vi "AP_project_calibration.vi"() -> ()   [LabVIEW 2019]
uses:
  <vilib>/userDefined/High Color/IMAQdx.ctl
  <vilib>/vision/driver/IMAQdx.llb/IMAQdx Acquisition Mode.ctl
  <vilib>/vision/driver/IMAQdx.llb/IMAQdx Buffer Number Mode.ctl
  <vilib>/vision/driver/NI_Vision_Acquisition_Software.lvlib
  <vilib>/vision/NI_Vision_Development_Module.lvlib
panel:
  in  "Range":cluster{"Lower value":sgl, "Upper value":sgl}={"Lower value"=50.0, "Upper value"=140.0} {"Upper value" format="%.2f"; "Lower value" format="%.2f"}
  out "DisplayFrameRate":dbl(knob) scale=0.0..100.0 scale format="%.1f"
  in  "IMAQdx Session":T1="cam0"
  out "ProcessBufferNumber":u32
  out "ProcessFrameRate":dbl(knob) scale=0.0..100.0 scale format="%.1f"
  out "Processed Image":T2(plugin-control)
  out "# elements in queue":i32(knob) scale=0.0..250.0
  in  "stop":bool
  out "CameraFrameRate":dbl(knob) scale=0.0..100.0 scale format="%.1f"
  out "CameraBuffer Number":u32
  out "Acquired Image":T2(plugin-control)
  out "height":dbl
  out "width":dbl
  in  "Display Index":i32
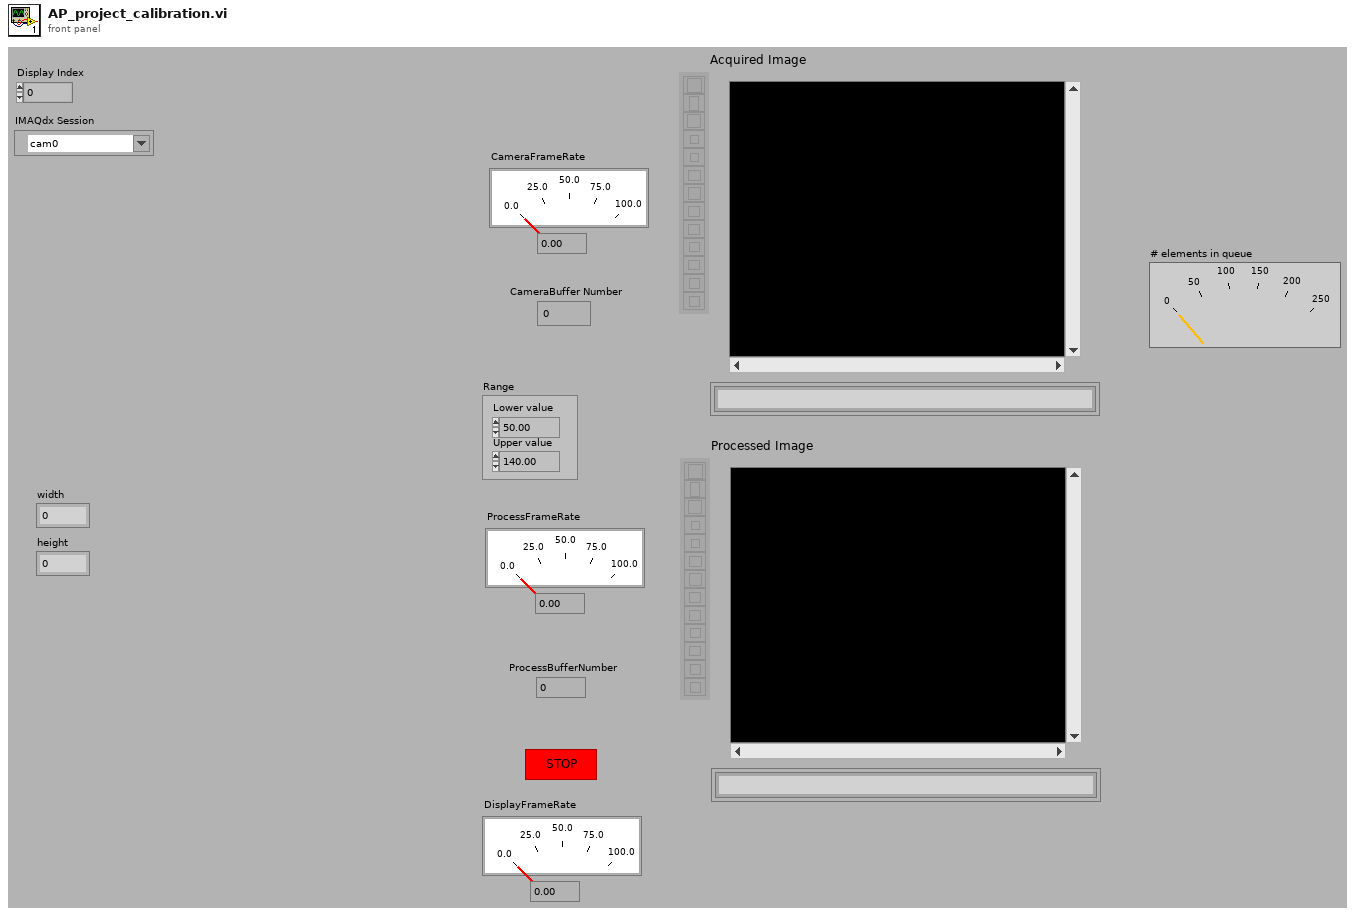
[diagram p1: front panel]
types:
  T1 = typedef "IMAQdx.ctl" = refnum<k21>
  T2 = typedef "IMAQ Image.ctl" = refnum<image>
  T3 = typedef "NI_Vision_Acquisition_Software.lvlib/IMAQdx Buffer Number Mode.ctl" = enum32{"Next", "Last", "Buffer Number", "Every", "Last New"}
  T4 = typedef "LVAllMonitorsDisplayTypeDef.ctl" = cluster{"Bounds":cluster{"Left":i16, "Top":i16, "Right":i16, "Bottom":i16}, "Depth":i16}[]
  T5 = cluster{"Bounds":cluster{"Left":i16, "Top":i16, "Right":i16, "Bottom":i16}, "Depth":i16}
  T6 = typedef "Image Type" = u32
  T7 = typedef "NI_Vision_Acquisition_Software.lvlib/IMAQdx Acquisition Mode.ctl" = enum32{"One Shot", "Continuous"}
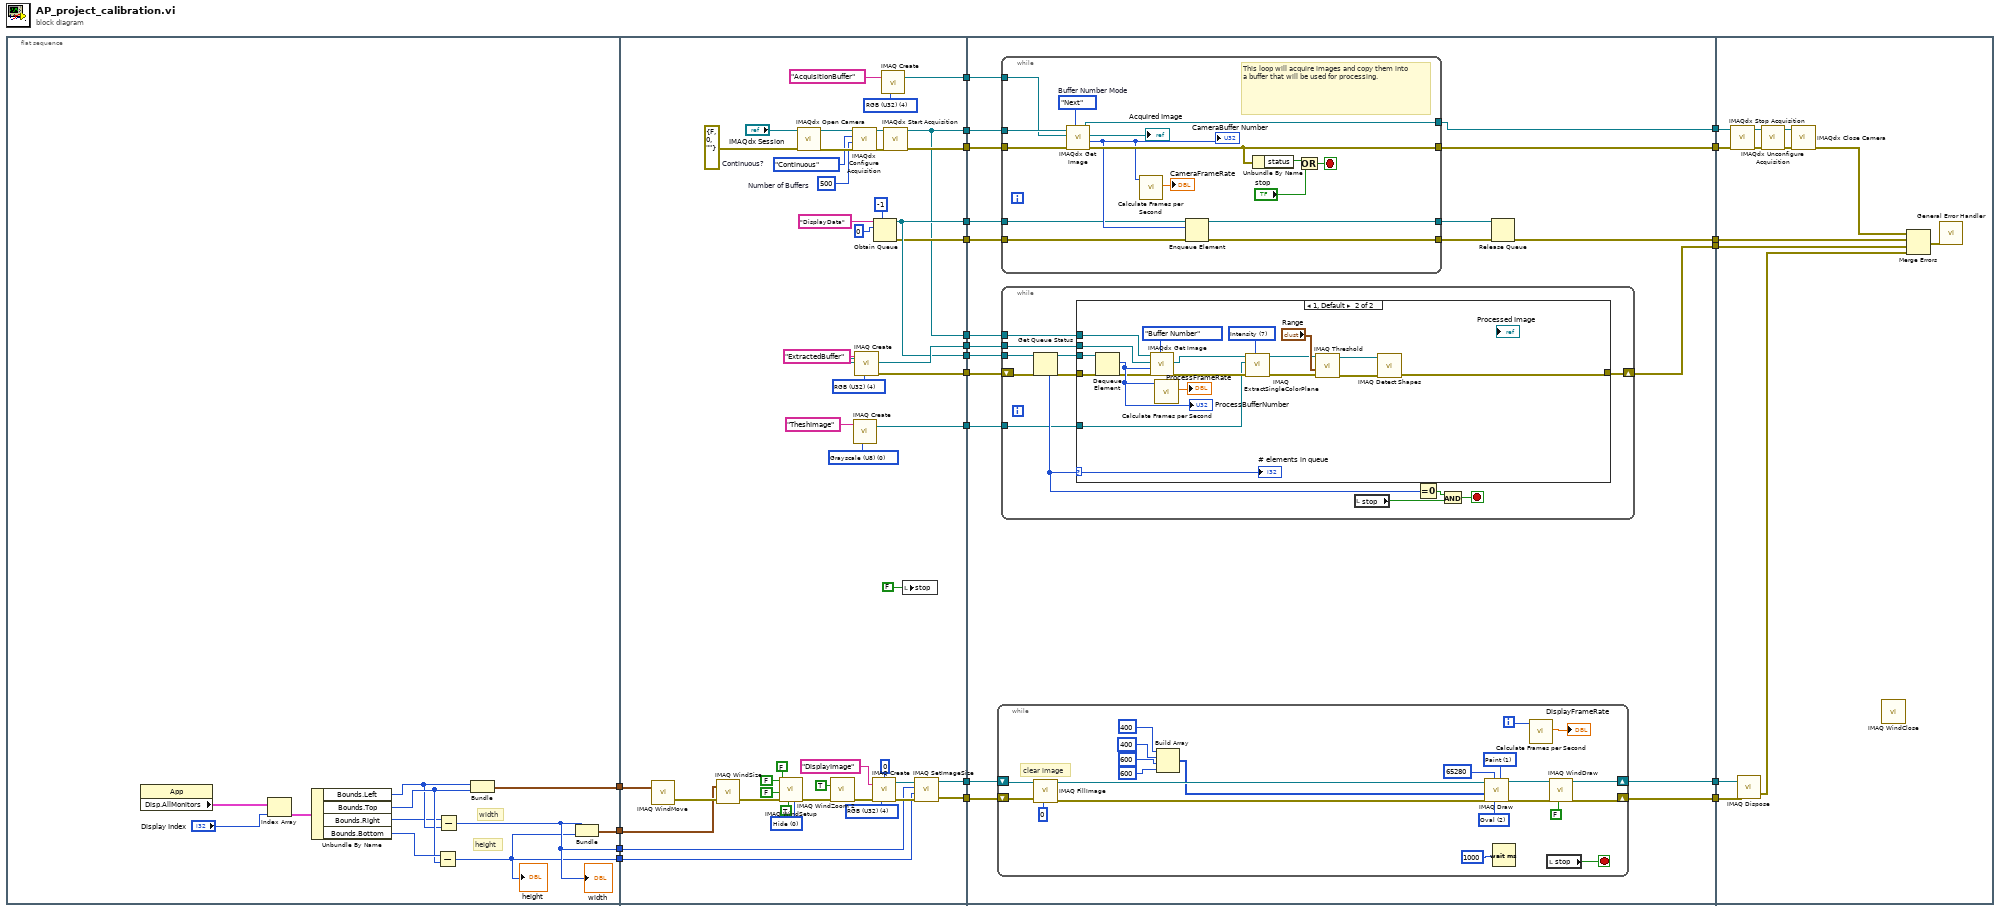
[diagram p0: block diagram]
diagram:
  n1 = flat-sequence {
    tunnel: [w26] -> w21
    tunnel: [w25] -> w20
    tunnel: [w24] -> w6
    tunnel: [w23] -> w5
    tunnel: [w45] -> w22
    tunnel: w21 -> [w77]
    tunnel: w20 -> [w75]
    tunnel: [w55] -> w19
    tunnel: [w54] -> w18
    tunnel: [w53] -> w17
    tunnel: [w53] -> w16
    tunnel: [w52] -> w15
    tunnel: [w51] -> w14
    tunnel: [w50] -> w9
    tunnel: [w50] -> w8
    tunnel: [w40] -> w7
    tunnel: w6 -> [w39]
    tunnel: w5 -> [w38]
    tunnel: [w37] -> w2
    tunnel: [w34] -> w1
    tunnel: w22 -> [w100]
    tunnel: w19 -> [w97]
    tunnel: w18 -> [w96]
    tunnel: w17 -> [w95]
    tunnel: w16 -> [w94]
    tunnel: w15 -> [w93]
    tunnel: w14 -> [w92]
    tunnel: [w91] -> w13
    tunnel: [w90] -> w12
    tunnel: [w89] -> w11
    tunnel: [w88] -> w10
    tunnel: w9 -> [w87]
    tunnel: w8 -> [w86]
    tunnel: w7 -> [w85]
    tunnel: [w84] -> w4
    tunnel: [w83] -> w3
    tunnel: w2 -> [w82]
    tunnel: w1 -> [w81]
    tunnel: w13 -> [w182]
    tunnel: w12 -> [w181]
    tunnel: w11 -> [w176]
    tunnel: w10 -> [w175]
    tunnel: w4 -> [w173]
    tunnel: w3 -> [w172]
    frame #0 {
      # "height"
      # "width"
      n2 = property class="App"() -> ("Disp.AllMonitors"=w29:T4)  [unwired: 2 in, 2 out]
      n3 = Index Array(array=w29, index="Display Index") -> (element=w28:T5)
      n4 = Unbundle By Name(w28) -> ("Bounds.Left"=w31:i16, "Bounds.Top"=w32:i16, "Bounds.Right"=w30:i16, "Bounds.Bottom"=w33:i16)
      n5 = Subtract(x=w33, y=w32) -> (x-y=w23:i16)
      "height" <- w23
      n6 = Subtract(x=w30, y=w31) -> (x-y=w24:i16)
      "width" <- w24
      n7 = Bundle("Left"=w31, "Top"=w32) -> (w25:cluster{"Left":i16, "Top":i16})  [unwired: 1 in]
      n8 = Bundle(w24, w23) -> (w26:cluster{i16, i16})  [unwired: 1 in]
    }
    frame #1 {
      w35 = T6 0 items=["Grayscale (U8)", "Grayscale (I16)", "Grayscale (SGL)", "Complex (CSG)", "RGB (U32)", "HSL (U32)", "RGB (U64)"] ("Image Type")
      w41 = T6 4 items=["Grayscale (U8)", "Grayscale (I16)", "Grayscale (SGL)", "Complex (CSG)", "RGB (U32)", "HSL (U32)", "RGB (U64)"] ("Image Type")
      w63 = T6 4 items=["Grayscale (U8)", "Grayscale (I16)", "Grayscale (SGL)", "Complex (CSG)", "RGB (U32)", "HSL (U32)", "RGB (U64)"] ("Image Type")
      w56 = T6 4 items=["Grayscale (U8)", "Grayscale (I16)", "Grayscale (SGL)", "Complex (CSG)", "RGB (U32)", "HSL (U32)", "RGB (U64)"] ("Image Type")
      w62 = u32 500  # Number of Buffers
      w61 = IMAQdx_Acquisition_Mode."Continuous"  # Continuous?
      w74 = 0 items=["Hide", "Show", "No change"] ("Scrollbars (No change)")
      n9 = call "IMAQ WindMove"("Coordinates (screen)"=w75) -> ("error out"=w79:errorcluster)  [unwired: 4 in, 1 out]
      n10 = call "IMAQ WindSize"("error in (no error)"=w79, "Width & Height"=w77) -> ("error out"=w80:errorcluster)  [unwired: 4 in, 2 out]
      n11 = call "IMAQ WindSetup"("Scrollbars (No change)"=w74, "Window is floating? (No)"=TRUE, "error in (no error)"=w80, "Window has title bar? (Yes)"=FALSE, "Window can close? (Yes)"=FALSE, "Window can grow? (Yes)"=FALSE) -> ("error out"=w78:errorcluster)  [unwired: 5 in]
      n12 = call <vilib>:"IMAQdx Open Camera.vi"("error in"=errorcluster {"status"=FALSE, "code"=0, "source"=""}, "Session In"="IMAQdx Session") -> ("error out"=w68:errorcluster, "Session Out"=w69:T1)  [unwired: 8 in]
      n13 = call "IMAQ WindZoom 2"("error in (no error)"=w78, "Zoom to Fit? (False)"=TRUE ("Zoom to Fit? (T)")) -> ("error out"=w44:errorcluster)  [unwired: 6 in, 3 out]
      n14 = call <vilib>:"IMAQdx Configure Acquisition.vi"("error in"=w68, "Number of Buffers"=w62, "Continuous?"=w61, "Session In"=w69) -> ("error out"=w67:errorcluster, "Session Out"=w65:T1)  [unwired: 6 in]
      n15 = call "IMAQ Create"("Image Name"="TheshImage", "Image Type"=w35) -> ("New Image"=w34:T2)  [unwired: 3 in, 1 out]
      n16 = call "IMAQ Create"("Image Name"="ExtractedBuffer", "Image Type"=w63) -> ("New Image"=w55:T2, "error out"=w37:errorcluster)  [unwired: 3 in]
      n17 = call "IMAQ Create"("Border Size"=0, "Image Name"="DisplayImage", "Image Type"=w41, "error in (no error)"=w44) -> ("New Image"=w46:T2, "error out"=w47:errorcluster)  [unwired: 1 in]
      n18 = Obtain Queue(max queue size (-1, unlimited)=-1, name (unnamed)="DisplayData", element data type=u32 0) -> (queue out=w53:refnum<queue>, error out=w52:errorcluster)  [unwired: 2 in, 1 out]
      n19 = call "IMAQ Create"("Image Name"="AcquisitionBuffer", "Image Type"=w56) -> ("New Image"=w51:T2)  [unwired: 3 in, 1 out]
      n20 = call <vilib>:"IMAQdx Start Acquisition.vi"("error in"=w67, "Session In"=w65) -> ("error out"=w54:errorcluster, "Session Out"=w50:T1)  [unwired: 8 in]
      n21 = local write "stop"(FALSE ("stop")) -> ()
      n22 = call "IMAQ SetImageSize"("error in (no error)"=w47, "Y Resolution"=w38, "X Resolution"=w39, "Image"=w46) -> ("error out"=w45:errorcluster, "Image Out"=w40:T2)  [unwired: 1 in]
    }
    frame #2 {
      n23 = while {
        shift-right: [w164] -> w84
        shift-left: w85 -> [w168]
        shift-right: [w163] -> w83
        shift-left: w100 -> [w167]
        i -> [w162]
        stop <- w169 stop-if-true
        w157 = u16 1 items=["Frame", "Paint", "Invert Frame", "Invert Paint"] ("Draw Mode")
        w156 = u16 2 items=["Line", "Rectangle", "Oval"] ("Shape to draw")
        # "clear image"
        n24 = call "IMAQ FillImage"("Color Pixel Value"=0, "error in (no error)"=w167, "Image"=w168) -> ("error out"=w158:errorcluster, "Image Out"=w154:T2)  [unwired: 7 in]
        n25 = Build Array(400, 400, 600, 600) -> (w153:i32[])
        n26 = call "IMAQ Draw"("Draw Mode"=w157, "Shape to draw"=w156, "Pixel Color"=65280, "error in (no error)"=w158, "Coordinates"=w153, "Image Src"=w154) -> ("error out"=w159:errorcluster, "Image Dst Out"=w160:T2)  [unwired: 4 in]
        n27 = Wait (ms)(milliseconds to wait=u32 1000) -> ()  [unwired: 1 out]
        n28 = call <vilib>:"Calculate Frames per Second.vi"("Buffer Number"=w162) -> ("Processed Frames/s"=→"DisplayFrameRate":dbl)  [unwired: 8 in, 2 out]
        n29 = local read "stop"() -> (w169:bool)
        n30 = call "IMAQ WindDraw"("Resize to Image Size? (Y)"=FALSE, "error in (no error)"=w159, "Image"=w160) -> ("error out"=w163:errorcluster, "Image Out (duplicate)"=w164:T2)  [unwired: 7 in]
      }
      n31 = while {
        tunnel: [w140] -> w89
        tunnel: [w145] -> w88
        tunnel: [w144] -> w98
        tunnel: [w143] -> w99
        tunnel: w96 -> [w137]
        tunnel: w94 -> [w135]
        tunnel: w93 -> [w134]
        tunnel: w92 -> [w133]
        tunnel: w87 -> [w136]
        stop <- w148 stop-if-true
        w142 = IMAQdx_Buffer_Number_Mode."Next"  # Buffer Number Mode
        # "This loop will acquire images and copy them into a buffer that will be used for processing."
        n32 = call <vilib>:"IMAQdx Get Image.vi"("Buffer Number Mode (Next)"=w142, "error in"=w137, "Image In"=w133, "Session In"=w136) -> ("error out"=w140:errorcluster, "Buffer Number Out"=w138:u32, "Image Out"=→"Acquired Image":T2, "Session Out"=w145:T1)  [unwired: 4 in]
        "CameraBuffer Number" <- w138
        n33 = call <vilib>:"Calculate Frames per Second.vi"("Buffer Number"=w138) -> ("Processed Frames/s"=→"CameraFrameRate":dbl)  [unwired: 8 in, 2 out]
        n34 = Enqueue Element(queue=w135, element=w138, error in (no error)=w134) -> (queue out=w144:refnum<queue>, error out=w143:errorcluster)  [unwired: 1 in, 1 out]
        n35 = Unbundle By Name(w140) -> ("status"=w147:bool)
        n36 = Or(x=w147, y="stop") -> (x .or. y?=w148:bool)
      }
      n37 = while {
        shift-right: [w111] -> w90
        shift-left: w82 -> [w103]
        tunnel: w97 -> [w110]
        tunnel: w86 -> [w109]
        tunnel: w95 -> [w108]
        tunnel: w81 -> [w101]
        stop <- w107 stop-if-true
        n38 = Get Queue Status(queue=w108, error in (no error)=w103) -> (queue out=w112:refnum<queue>, error out=w102:errorcluster, # elements in queue=w104:i32)  [unwired: 1 in, 5 out]
        n39 = case shown="1, Default" w104 {
          selector: w104 -> [_ w128]
          tunnel: w112 -> [_ w132]
          tunnel: w110 -> [_ w129]
          tunnel: [w113 w116] -> w111
          tunnel: w109 -> [_ w131]
          tunnel: w102 -> [w113 w119]
          tunnel: w101 -> [_ w117]
          frame 0 {
          }
          frame 1, Default {
            w124 = 7 items=["Red", "Green", "Blue", "Hue", "Saturation", "Luminance", "Value", "Intensity"] ("Color Plane")
            n40 = Dequeue Element(queue=w132, error in (no error)=w119) -> (element=w127:u32, error out=w118:errorcluster)  [unwired: 1 in, 2 out]
            "ProcessBufferNumber" <- w127
            n41 = call <vilib>:"IMAQdx Get Image.vi"("Buffer Number Mode (Next)"=IMAQdx_Buffer_Number_Mode."Buffer Number", "error in"=w118, "Buffer Number In"=w127, "Image In"=w129, "Session In"=w131) -> ("error out"=w121:errorcluster, "Image Out"=w122:T2)  [unwired: 3 in, 2 out]
            n42 = call <vilib>:"Calculate Frames per Second.vi"("Buffer Number"=w127) -> ("Processed Frames/s"=→"ProcessFrameRate":dbl)  [unwired: 8 in, 2 out]
            n43 = call "IMAQ ExtractSingleColorPlane"("Color Plane"=w124, "error in (no error)"=w121, "Image Dst"=w117, "Image Src"=w122) -> ("error out"=w120:errorcluster, "Image Dst Out"=w123:T2)  [unwired: 6 in]
            n44 = call "IMAQ Threshold"("error in (no error)"=w120, "Range"="Range", "Image Src"=w123) -> ("error out"=w115:errorcluster, "Image Dst Out"=w114:T2)  [unwired: 7 in]
            n45 = call-poly "IMAQ Detect Shapes"("error in (no error)"=w115, "Image"=w114) -> ("error out"=w116:errorcluster)  [unwired: 7 in, 2 out]
            "# elements in queue" <- w128
          }
        }
        n46 = local read "stop"() -> (w106:bool)
        n47 = Equal To 0?(x=w104) -> (x = 0?=w105:bool)
        n48 = And(x=w105, y=w106) -> (x .and. y?=w107:bool)
      }
      n49 = Release Queue(queue=w98, error in (no error)=w99) -> (error out=w91:errorcluster)  [unwired: 1 in, 2 out]
    }
    frame #3 {
      n50 = call <vilib>:"IMAQdx Stop Acquisition.vi"("error in"=w176, "Session In"=w175) -> ("error out"=w177:errorcluster, "Session Out"=w178:T1)  [unwired: 8 in]
      n51 = call "IMAQ Dispose"("Image"=w173, "error in (no error)"=w172) -> ("error out"=w171:errorcluster)  [unwired: 4 in]
      n52 = call <vilib>:"IMAQdx Unconfigure Acquisition.vi"("error in"=w177, "Session In"=w178) -> ("error out"=w180:errorcluster, "Session Out"=w179:T1)  [unwired: 8 in]
      n53 = call <vilib>:"IMAQdx Close Camera.vi"("error in"=w180, "Session In"=w179) -> ("error out"=w174:errorcluster)  [unwired: 9 in]
      n54 = call "IMAQ WindClose"() -> ()  [unwired: 6 in, 1 out]
      n55 = Merge Errors(w174, w182, w181, w171) -> (w183:errorcluster)
      n56 = call <vilib>:"General Error Handler.vi"("error in (no error)"=w183) -> ()  [unwired: 10 in, 5 out]
    }
  }
